vi "Set Destination.vi"(8 "error in (no error)":errorcluster, 9 "Destination label":string, 10 "ProjectItem Refnum":refnum<vi>, 11 "SDIST in":refnum<class "NI_AB_API_SDIST.lvclass">) -> (0 "error out":errorcluster, 3 "SDIST out":refnum<class "NI_AB_API_SDIST.lvclass">)   [LabVIEW 2020, in "NI_AB_API_SDIST.lvclass"]
uses:
  <vilib>/AppBuilder/AB_API/SDIST/NI_AB_API_SDIST.lvclass
  <vilib>/AppBuilder/AB_API/Build/NI_AB_API_Build.lvclass
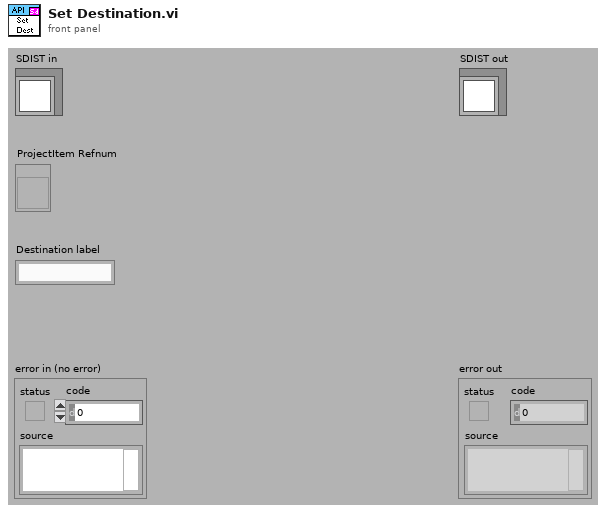
[diagram p1: front panel]
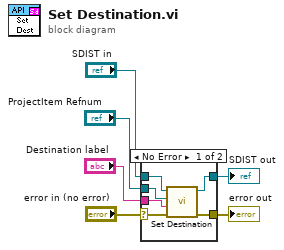
[diagram p0: block diagram]
diagram:
  n1 = case shown="No Error" "error in (no error)" {
    selector: "error in (no error)" -> [w9 w14]
    tunnel: [w10 w14] -> w5
    tunnel: [w11 w13] -> w3
    tunnel: "SDIST in" -> [w12 w13]
    tunnel: "ProjectItem Refnum" -> [w8 _]
    tunnel: "Destination label" -> [w7 _]
    frame No Error {
      n2 = call-parent "Set Destination.vi"("error in (no error)"=w9, "Destination label"=w7, "ProjectItem Refnum"=w8, "Build in"=w12) -> ("error out"=w10:errorcluster, "Build out"=w11:refnum<class "NI_AB_API_SDIST.lvclass">)  [unwired: 6 in]
    }
    frame Error {
    }
  }
  "error out" <- w5
  "SDIST out" <- w3
